vi "Read optical zero.vi"(8 "error in (no error)":errorcluster, 11 "Control-Client in":refnum<class "Control-Client.lvclass">) -> (0 "error out":errorcluster, 2 "optical zero":dbl, 3 "Control-Client out":refnum<class "Control-Client.lvclass">)   [LabVIEW 2020, in "Control-Client.lvclass"]
uses:
  Control-Client.lvclass
  Control-Client.lvclass/Control-Client.ctl
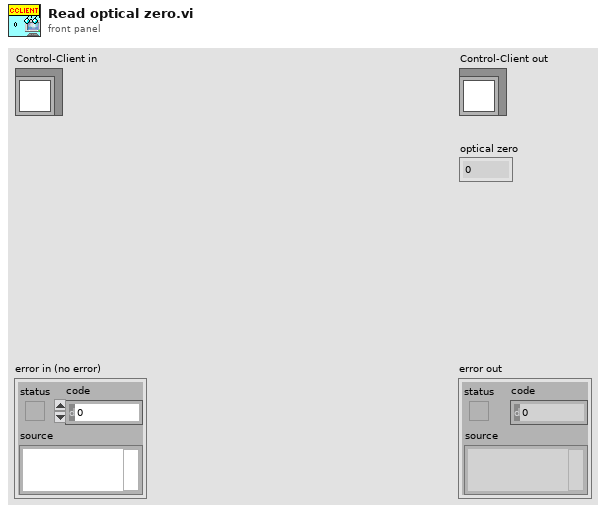
[diagram p1: front panel]
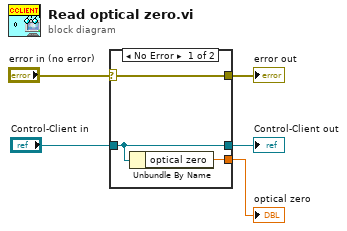
[diagram p0: block diagram]
diagram:
  n1 = case shown="No Error" "error in (no error)" {
    selector: "error in (no error)" -> [w8 w9]
    tunnel: [w8 w9] -> w4
    tunnel: [w7 w10] -> w2
    tunnel: "Control-Client in" -> [w7 w10]
    tunnel: [w6 _] -> w1
    frame No Error {
      n2 = Unbundle By Name(w7) -> ("optical zero"=w6:dbl)
    }
    frame Error {
    }
  }
  "error out" <- w4
  "Control-Client out" <- w2
  "optical zero" <- w1
